vi "Top_Level_Control_v00.vi"() -> ()   [LabVIEW 2010]
uses:
  <vilib>/rvi/interface/nirviCloseFPGA/nirviCloseFPGA.xnode
  <vilib>/rvi/interface/nirviOpenFPGA/nirviOpenFPGA.xnode
  <vilib>/userDefined/High Color/nirio_resource_hc.ctl
  <vilib>/rvi/interface/nirviReadWriteControl/nirviReadWriteControl.xnode
  <vilib>/Utility/error.llb/Error Cluster From Error Code.vi
  <vilib>/rvi/interface/nirviMethod/nirviMethod.xnode
  <vilib>/FPGAPlugInAG/Dynamic/niLvFpga_Close_Dynamic.vi
  NiFpgaLv.dll
  Temporal Clusters Control/FPGA Bitfiles/TemporalClusters_FPGABSlot3_GraphFPGAv07_B46A369A.lvbitx
  Program Files/National Instruments/LabVIEW 2010/Targets/NI/FPGA/StockFPGA_IntfPrivate/ScriptTemplates/StockFPGA_ReadBigControlPlusUnflatten.vi
  Program Files/National Instruments/LabVIEW 2010/Targets/NI/FPGA/StockFPGA_IntfPrivate/ScriptTemplates/StockFPGA_FlattenPlusWriteBigControl.vi
  Program Files/National Instruments/LabVIEW 2010/Targets/NI/FPGA/StockFPGA_IntfPrivate/ScriptTemplates/StockFPGA_InlinedAdjustErrorForReadWrite.vi
  FPGA Bitfiles/PIIphaselocks_FPGATarget_CavitiesPulseFPG_483F4CC6.lvbitx
  <vilib>/FPGAPlugInAG/PXI-7833R/niLvFpga_Open_PXI-7833R.vi
  <vilib>/rvi/ClientSDK/nirviWhatTheDeviceIsDoing.ctl
  <vilib>/rvi/interface/common/dynamic/niFpgaDynamicAddResources.vi
  <vilib>/rvi/errors/niLvFpgaWhatHappensToTopLevelVI.ctl
  <vilib>/rvi/interface/common/niFpgaNodeNameForErrorReporting.ctl
  <vilib>/rvi/errors/niLvFpgaAdjustHostInterfaceError.vi
  Strict Type Defs/Lock or Hold.ctl
  Strict Type Defs/Slider and display.ctl
  Strict Type Defs/I16 white control.ctl
  Strict Type Defs/PII Gains.ctl
  Strict Type Defs/DC polarity.ctl
  Strict Type Defs/Thresh slider.ctl
  Strict Type Defs/I2 gain slider.ctl
  Strict Type Defs/Scan Freq Slider.ctl
  Strict Type Defs/Gains negative vertical.ctl
  Strict Type Defs/Control GUI v01.ctl
  Strict Type Defs/Lock Select.ctl
  Strict Type Defs/Hold All.ctl
  Strict Type Defs/Scope and Safety.ctl
  Strict Type Defs/Pre-Offset.ctl
  Strict Type Defs/Cavity Extras.ctl
  Strict Type Defs/Pulse Control.ctl
  Strict Type Defs/theta.ctl
  Strict Type Defs/Control GUI Graph v00.ctl
  Strict Type Defs/Graph Extras.ctl
  Strict Type Defs/Double Graph control.ctl
  Strict Type Defs/I16 Graph Control.ctl
  Strict Type Defs/GUI HD Graph.ctl
panel:
  out "Any Unlocked?":bool=TRUE
  out "Locked?":T1={"OPO A"=FALSE, "OPO B"=FALSE, "MCC"=FALSE, "Doubler"=TRUE}
  out "Locked?(Graph)":T2={"パラメ A"=TRUE, "パラメ B"=TRUE, "EPR BS"=TRUE, "Graph BS"=TRUE, "HD A"=TRUE, "HD B"=TRUE}
  in  "Measurement OFF":bool
  in  "watertank":bool
  out "Water Tank":dbl(slide)=-0.29411764705882354 scale=-0.3..0.3
  in  "Stop Pulses":bool
  in  "Pulses":bool
  out "Top Loop Count":i32=272090
  out "Measurment Pulse":bool
  out "HD Pulse":bool
  out "Probe OFF Pulse":bool=TRUE
  out "BS Hold Pulse":bool=TRUE
  in  "stop":bool
  in  "Hold All":T3
  in  "Extra Controls":T4(tab)=enum."Other"
  in  "Scope+Safety":T5={"Safety First"={"lim reset"=FALSE, "no limit"=FALSE, "pos slew rate * dt"=12, "neg slew rate * dt"=-12, "Count(Ticks)"=0}, "Scope IPs"={"Trigger Direction"=enum."minus-plus", "Trigger Delay (ms)"=0.0, "Aquisition Rate (kHz)"=4000.0, "Trigger Offset (V)"=0.0, "Scale Offset"={"Scaling"={"Error signal"=1, "Output"=0, "DC Monitor"=1, "Threshold"=1}, "Offset"={"Error Signal"=0, "Output"=0, "DC Monitor"=0, "Threshold"=0}}}}
  in  "Graph Extras":T6={"Error Bit Sh."={"パラメ A"=-2, "パラメ B"=-2, "EPR BS"=0, "Graph BS"=0, "HD A x"=-2, "HD A p"=-2, "HD B x"=-4, "HD B p"=-3}, "I Max value"=2147483647, "I2 Max value"=2147483647, "Scan Offset"={"パラメ A"=0.0, "パラメ B"=0.0, "EPR BS"=0.0, "Graph BS"=0.0, "HD A"=0.0, "HD B"=0.0}, "Scan Ampl."={"パラメ A"=1000.0, "パラメ B"=1000.0, "EPR BS"=1200.0, "Graph BS"=100.0, "HD A"=2000.0, "HD B"=2000.0}, "Scan-PII thresh"={"パラメ A"=100, "パラメ B"=100, "EPR BS"=100, "Graph BS"=100, "Homodyne A"=100, "Homodyne B"=100}, "Re-Scan thresh"={"パラメ A"=1, "パラメ B"=1, "EPR BS"=1, "Graph BS"=1, "Homodyne A"=1, "Homodyne B"=1}, "Post-Offset"={"HD A x"=0.0, "HD A p"=0.0, "HD B x"=0.0, "HD B p"=0.0}}
  in  "Cavity Extras":T9={"Pre-Offset"={"OPO A"=0.0, "OPO B"=0.0, "MCC"=0.0, "Doubler"=0.0}, "Pre-Offset DC"={"OPO A"=0.0, "OPO B"=0.0, "MCC"=0.0, "Doubler"=0.0}, "I Max value"=2147483647, "I2 Max value"=0, "Scan Offset"={"OPO A"=0.0, "OPO B"=0.0, "MCC"=0.0, "Doubler"=0.0}, "Scan Ampl."={"OPO A"=1000.0, "OPO B"=1000.0, "MCC"=1000.0, "Doubler"=1000.0}, "Scan-PII thresh"={"OPO A"=100, "OPO B"=100, "MCC"=100, "Doubler"=100}, "Re-Scan thresh"={"OPO A"=1, "OPO B"=1, "MCC"=4, "Doubler"=0}}
  out "xy HD A":cluster{i16[], i16[]}(graph)
  in  "XY HD ON":bool
  out "xy HD B":cluster{i16[], i16[]}(graph)
  in  "Pulse Control":T11={"BS Hold Invert"=FALSE, "Probe Invert"=FALSE, "HD Invert"=TRUE, "Measurement Invert"=FALSE, "BS Hold Delay"=0, "Probe Delay"=10, "HD Delay"=25, "Measurement delay"=80, "High Pulse"=4000, "Low Pulse"=-3200, "Sample & Hold Period (uSec)"=500, "BS Hold ON until"=325, "Probe OFF until"=315, "HD ON until"=305, "Measurement ON until"=280, "Loop period (us)"=0}
  in  "RMS Thresh":T12={"Pump A"=40, "Pump B"=40, "EPR"=40, "Graph"=40, "HD A"=40, "HD B"=40}
  out "Cavities Pulse Loop count":i32=247262374
  out "Tick Count Cavities (uSec)":u32=4069594290 caption="Cavities Tick Count (uSec)"
  out "Cavities Control Loop count":i32=2147483647
  in  "Safety First Graph":T13={"lim reset"=FALSE, "no limit"=FALSE, "pos slew rate * dt"=40, "neg slew rate * dt"=-40, "Count(Ticks)"=0}
  out "Measurement Tick Count(uSec)":u32=500
  in  "offset time":u32=100
  in  "Measurement OFF (uSec)":u32=1100000
  in  "Inverse (Graph)":bool
  out "PXI Trig 1":bool
  in  "Lock Monitor":T14={"OPO A"=80, "OPO B"=80, "MCC"=80, "Doubler"=0}
  out "PXI Trig 2":bool=TRUE
  out "Cavities error out":errorcluster
  out "Graph error":errorcluster
  in  "Loop Delays (uSec)":u32=5
  in  "Number of Elements":u32=4095
  in  "Cavities_FPGA_v07":T15="RIO0" caption="RIO Device"
  in  "Graph_FPGA_v07":T15="RIO1" caption="RIO Device"
  in  "Scope":T16=TRUE
  out "Scope Graph":cluster{dbl[], dbl[]}[](graph)
  in  "Lock Select":T17
  in  "OPO A":T18={"Offset Error"=-0.004322033898305084, "Gain Error"=1, "Offset DC"=0.18926553672316412, "Gain DC"=1, "P Gain"=12, "P Bit Shift"=-7, "I Bit Shift"=-7, "I2 Bit Shift"=-27, "I Gain"=19, "I2 Gain"=0, "Lock Threshold"=66, "Lock"=FALSE, "Hold"=FALSE, "Scan Frequency"=19, "Scan Bit Shift"=-4, "DC negative"=FALSE, "Gains -ve "=FALSE} {"Scan Frequency" scale=1.0..30.0; "I2 Gain" scale=0.0..10.0; "I Gain" scale=0.0..50.0; "P Gain" scale=0.0..50.0; "Offset DC" scale=-5.0..0.5 scale format="%#_5f"; "Offset Error" scale=-0.01..0.005 scale format="%#_5f"}
  in  "OPO B":T18={"Offset Error"=-0.011977401129943503, "Gain Error"=4, "Offset DC"=1.29177966101695, "Gain DC"=1, "P Gain"=14, "P Bit Shift"=-8, "I Bit Shift"=-8, "I2 Bit Shift"=-27, "I Gain"=13, "I2 Gain"=0, "Lock Threshold"=67, "Lock"=FALSE, "Hold"=FALSE, "Scan Frequency"=10, "Scan Bit Shift"=-5, "DC negative"=TRUE, "Gains -ve "=FALSE} {"Scan Frequency" scale=1.0..30.0; "I2 Gain" scale=0.0..10.0; "I Gain" scale=0.0..50.0; "P Gain" scale=0.0..50.0; "Offset DC" scale=-5.1..3.0 scale format="%#_5f"; "Offset Error" scale format="%#_5f"}
  in  "MCC":T18={"Offset Error"=-0.006610169491525424, "Gain Error"=1, "Offset DC"=0.028813559322033905, "Gain DC"=1, "P Gain"=14, "P Bit Shift"=-8, "I Bit Shift"=-11, "I2 Bit Shift"=-27, "I Gain"=11, "I2 Gain"=0, "Lock Threshold"=20, "Lock"=FALSE, "Hold"=FALSE, "Scan Frequency"=10, "Scan Bit Shift"=-4, "DC negative"=TRUE, "Gains -ve "=TRUE} {"Scan Frequency" scale=1.0..30.0; "I2 Gain" scale=0.0..10.0; "I Gain" scale=0.0..50.0; "P Gain" scale=0.0..50.0; "Offset DC" scale=-0.1..0.2 scale format="%#_5f"; "Offset Error" scale=-0.02..0.01 scale format="%#_5f"}
  in  "Doubler":T18={"Offset Error"=-0.011581920903954804, "Gain Error"=1, "Offset DC"=-0.023163841807909608, "Gain DC"=1, "P Gain"=10, "P Bit Shift"=-7, "I Bit Shift"=-8, "I2 Bit Shift"=-27, "I Gain"=21, "I2 Gain"=0, "Lock Threshold"=12, "Lock"=FALSE, "Hold"=FALSE, "Scan Frequency"=8, "Scan Bit Shift"=-5, "DC negative"=FALSE, "Gains -ve "=FALSE} {"Scan Frequency" scale=1.0..30.0; "I2 Gain" scale=0.0..10.0; "I Gain" scale=0.0..50.0; "P Gain" scale=0.0..50.0; "Offset DC" scale=-0.1..0.1 scale format="%#_5f"; "Offset Error" scale=-0.05..0.05 scale format="%#_5f"}
  in  "パラメ A":T27={"Offset Error"=-0.004689265536723164, "Gain Error"=2, "P Gain"=10, "P Bit Shift"=-7, "I Bit Shift"=-9, "I2 Bit Shift"=-27, "I Gain"=12, "I2 Gain"=0, "Lock Threshold"=13, "Lock"=FALSE, "Hold"=TRUE, "Scan Frequency"=12, "Scan Bit Shift"=-6, "Gains -ve "=FALSE, "Pre- Offset Error"=0.00367231638418079} {"Pre- Offset Error" scale=-0.05..0.05 scale format="%#_5f"; "Scan Frequency" scale=1.0..30.0; "I2 Gain" scale=0.0..10.0; "I Gain" scale=0.0..50.0; "P Gain" scale=0.0..50.0; "Offset Error" scale=-0.01..0.01 scale format="%#_5f"}
  in  "パラメ B":T27={"Offset Error"=0.003389830508474575, "Gain Error"=1, "P Gain"=31, "P Bit Shift"=-8, "I Bit Shift"=-9, "I2 Bit Shift"=-16, "I Gain"=20, "I2 Gain"=3, "Lock Threshold"=13, "Lock"=FALSE, "Hold"=TRUE, "Scan Frequency"=6, "Scan Bit Shift"=-5, "Gains -ve "=FALSE, "Pre- Offset Error"=0.02768361581920904} {"Pre- Offset Error" scale=-0.1..0.1 scale format="%#_5f"; "Scan Frequency" scale=1.0..30.0; "I2 Gain" scale=0.0..10.0; "I Gain" scale=0.0..50.0; "P Gain" scale=0.0..50.0; "Offset Error" scale=-0.04..0.04 scale format="%#_5f"}
  in  "EPR BS":T27={"Offset Error"=-0.0003333333333333334, "Gain Error"=1, "P Gain"=25, "P Bit Shift"=-10, "I Bit Shift"=-10, "I2 Bit Shift"=-17, "I Gain"=22, "I2 Gain"=3, "Lock Threshold"=14, "Lock"=FALSE, "Hold"=TRUE, "Scan Frequency"=9, "Scan Bit Shift"=-6, "Gains -ve "=FALSE, "Pre- Offset Error"=0.011468926553672315} {"Pre- Offset Error" scale=-0.01..0.03 scale format="%#_5f"; "Scan Frequency" scale=1.0..30.0; "I2 Gain" scale=0.0..10.0; "I Gain" scale=0.0..50.0; "P Gain" scale=0.0..50.0; "Offset Error" scale=-0.001..0.001 scale format="%#_5f"}
  in  "Graph BS":T27={"Offset Error"=-0.0011751412429378532, "Gain Error"=1, "P Gain"=12, "P Bit Shift"=-7, "I Bit Shift"=-10, "I2 Bit Shift"=-16, "I Gain"=15, "I2 Gain"=3, "Lock Threshold"=13, "Lock"=FALSE, "Hold"=TRUE, "Scan Frequency"=7, "Scan Bit Shift"=-5, "Gains -ve "=FALSE, "Pre- Offset Error"=0.012796610169491527} {"Pre- Offset Error" scale=-0.005..0.02 scale format="%#_5f"; "Scan Frequency" scale=1.0..30.0; "I2 Gain" scale=0.0..10.0; "I Gain" scale=0.0..50.0; "P Gain" scale=0.0..50.0; "Offset Error" scale format="%#_5f"}
  in  "Homodyne A":T28={"Pre-Offset p Error"=-0.027683615819209043, "Gain Error x"=2, "P Gain"=13, "P Bit Shift"=-10, "I Bit Shift"=-8, "I2 Bit Shift"=-11, "I Gain"=22, "I2 Gain"=2, "Lock Threshold"=28, "Lock"=FALSE, "Hold"=TRUE, "Scan Frequency"=10, "Scan Bit Shift"=-5, "Gains -ve "=FALSE, "Pre- Offset x"=0.02768361581920904, "Lock Angle (θ)"=90.0, "Gain Error p\n\n"=1} {"Lock Angle (θ)" min=-90.0 max=90.0 scale=-90.0..90.0 scale format="%#_2g"; "Pre- Offset x" scale=-0.1..0.1 scale format="%#_5f"; "Scan Frequency" scale=1.0..30.0; "I2 Gain" scale=0.0..10.0; "I Gain" scale=0.0..50.0; "P Gain" scale=0.0..50.0; "Pre-Offset p Error" scale=-0.1..0.1 scale format="%#_5f"}
  in  "Homodyne B":T28={"Pre-Offset p Error"=0.015536723163841807, "Gain Error x"=1, "P Gain"=20, "P Bit Shift"=-6, "I Bit Shift"=-5, "I2 Bit Shift"=-15, "I Gain"=12, "I2 Gain"=3, "Lock Threshold"=15, "Lock"=FALSE, "Hold"=TRUE, "Scan Frequency"=7, "Scan Bit Shift"=-5, "Gains -ve "=TRUE, "Pre- Offset x"=-0.011864406779661014, "Lock Angle (θ)"=90.0, "Gain Error p\n\n"=5} {"Lock Angle (θ)" min=-90.0 max=90.0 scale=-90.0..90.0 scale format="%#_2g"; "Pre- Offset x" scale=-0.1..0.05 scale format="%#_5f"; "Scan Frequency" scale=1.0..30.0; "I2 Gain" scale=0.0..10.0; "I Gain" scale=0.0..50.0; "P Gain" scale=0.0..50.0; "Pre-Offset p Error" scale=-0.05..0.05 scale format="%#_5f"}
  # "All time values are in micro-seconds"
  # "PII Gains"
  # "Lock"
  # "Error Signal"
  # "Monitor"
  # "Scan"
  # "DC positive"
  # "PII Gains"
  # "Lock"
  # "Error Signal"
  # "Monitor"
  # "Scan"
  # "DC positive"
  # "PII Gains"
  # "Lock"
  # "Error Signal"
  # "Monitor"
  # "Scan"
  # "DC positive"
  # "PII Gains"
  # "Lock"
  # "Error Signal"
  # "Monitor"
  # "Scan"
  # "DC positive"
  # "PII Gains"
  # "Lock"
  # "Error Signal"
  # "Scan"
  # "PII Gains"
  # "Lock"
  # "Error Signal"
  # "Scan"
  # "PII Gains"
  # "Lock"
  # "Error Signal"
  # "Scan"
  # "PII Gains"
  # "Lock"
  # "Error Signal"
  # "Scan"
  # "PII Gains"
  # "Lock"
  # "Error Signal"
  # "Scan"
  # "PII Gains"
  # "Lock"
  # "Error Signal"
  # "Scan"
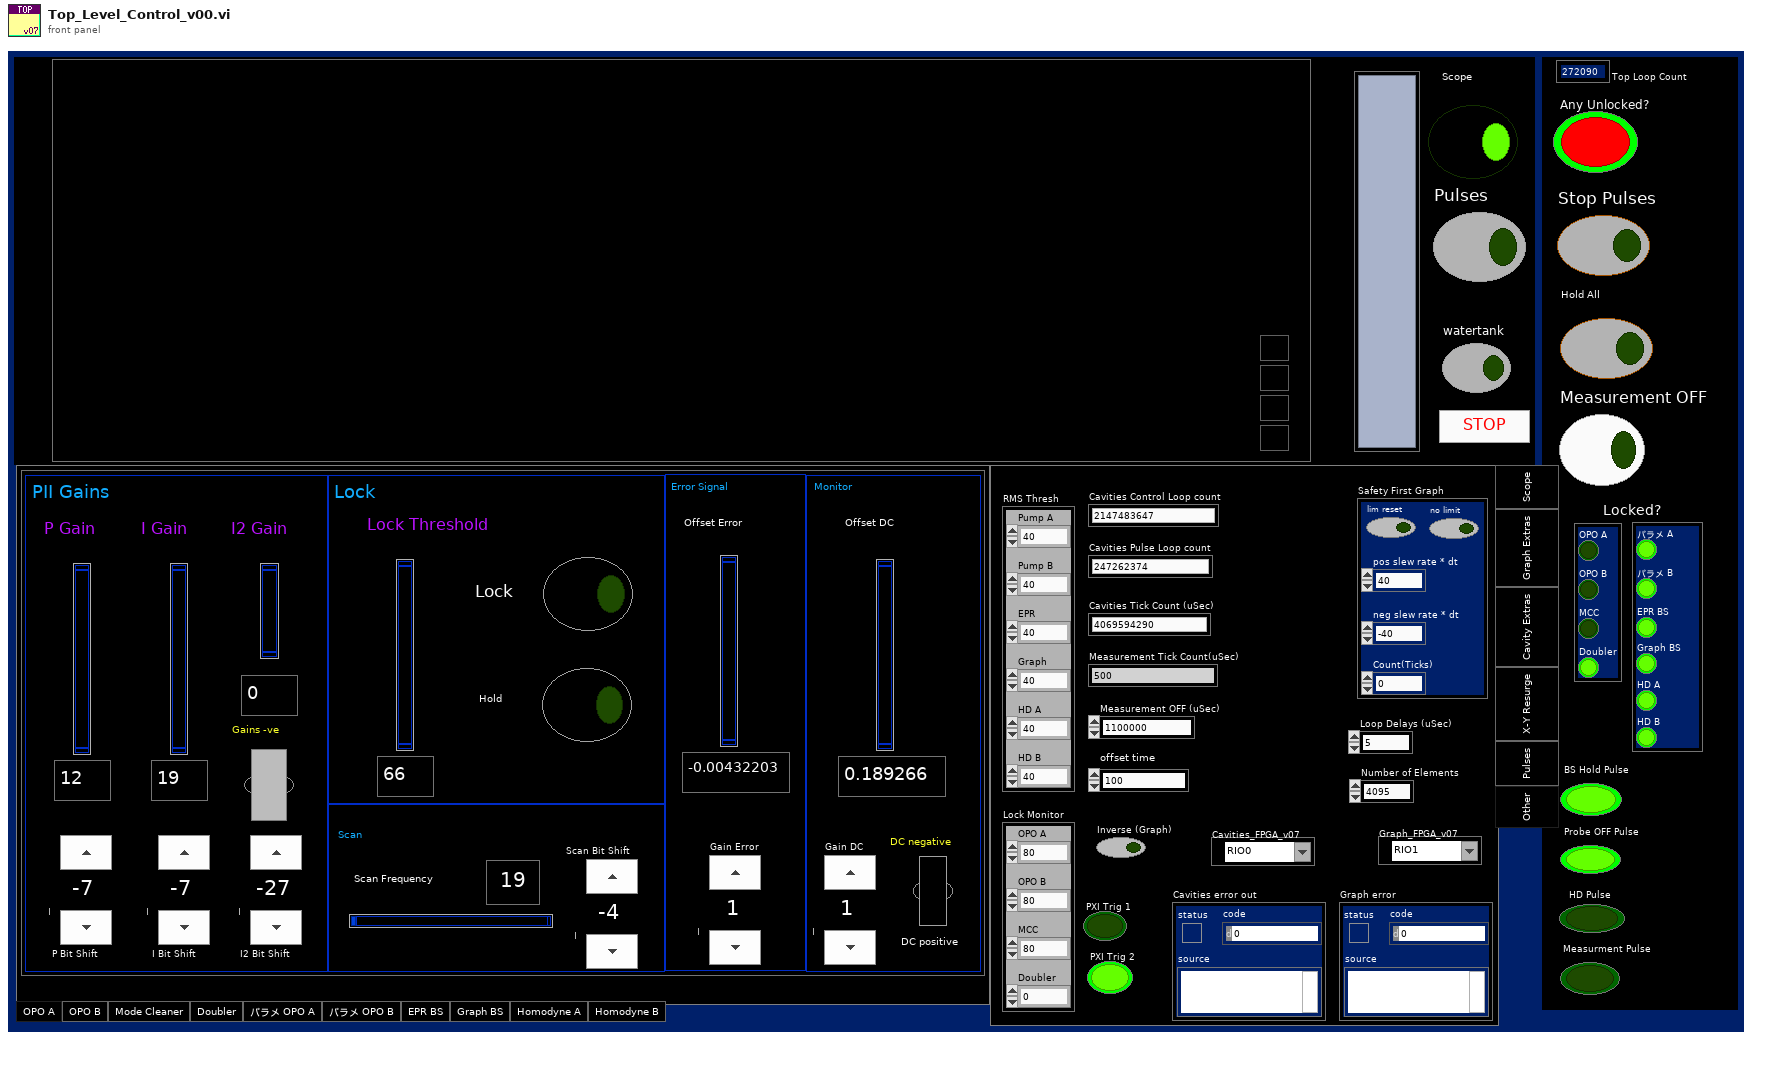
[diagram p1: front panel]
types:
  T1 = cluster{"OPO A":bool, "OPO B":bool, "MCC":bool, "Doubler":bool}
  T2 = cluster{"パラメ A":bool, "パラメ B":bool, "EPR BS":bool, "Graph BS":bool, "HD A":bool, "HD B":bool}
  T3 = typedef "Hold All.ctl" = bool
  T4 = enum32{"Scope", "Graph Extras", "Cavity Extras", "X-Y Resurge", "Pulses", "Other"}
  T5 = typedef "Scope and Safety.ctl" = cluster{"Safety First":cluster{"lim reset":bool, "no limit":bool, "pos slew rate * dt":i16, "neg slew rate * dt":i16, "Count(Ticks)":u32}, "Scope IPs":cluster{"Trigger Direction":enum8{"either", "minus-plus", "plus-minus"}, "Trigger Delay (ms)":dbl, "Aquisition Rate (kHz)":dbl, "Trigger Offset (V)":dbl, "Scale Offset":cluster{"Scaling":cluster{"Error signal":i16, "Output":i16, "DC Monitor":i16, "Threshold":i16}, "Offset":cluster{"Error Signal":i16, "Output":i16, "DC Monitor":i16, "Threshold":i16}}}}
  T6 = typedef "Graph Extras.ctl" = cluster{"Error Bit Sh.":cluster{"パラメ A":i16, "パラメ B":i16, "EPR BS":i16, "Graph BS":i16, "HD A x":i16, "HD A p":i16, "HD B x":i16, "HD B p":i16}, "I Max value":i32, "I2 Max value":i32, "Scan Offset":T7, "Scan Ampl.":T7, "Scan-PII thresh":T8, "Re-Scan thresh":T8, "Post-Offset":cluster{"HD A x":dbl, "HD A p":dbl, "HD B x":dbl, "HD B p":dbl}}
  T7 = typedef "Double Graph control.ctl" = cluster{"パラメ A":dbl, "パラメ B":dbl, "EPR BS":dbl, "Graph BS":dbl, "HD A":dbl, "HD B":dbl}
  T8 = typedef "I16 Graph Control.ctl" = cluster{"パラメ A":i16, "パラメ B":i16, "EPR BS":i16, "Graph BS":i16, "Homodyne A":i16, "Homodyne B":i16}
  T9 = typedef "Cavity Extras.ctl" = cluster{"Pre-Offset":T10, "Pre-Offset DC":T10, "I Max value":i32, "I2 Max value":i32, "Scan Offset":T10, "Scan Ampl.":T10, "Scan-PII thresh":cluster{"OPO A":i16, "OPO B":i16, "MCC":i16, "Doubler":i16}, "Re-Scan thresh":cluster{"OPO A":i16, "OPO B":i16, "MCC":i16, "Doubler":i16}}
  T10 = typedef "Pre-Offset.ctl" = cluster{"OPO A":dbl, "OPO B":dbl, "MCC":dbl, "Doubler":dbl}
  T11 = typedef "Pulse Control.ctl" = cluster{"BS Hold Invert":bool, "Probe Invert":bool, "HD Invert":bool, "Measurement Invert":bool, "BS Hold Delay":u32, "Probe Delay":u32, "HD Delay":u32, "Measurement delay":u32, "High Pulse":i16, "Low Pulse":i16, "Sample & Hold Period (uSec)":u32, "BS Hold ON until":u32, "Probe OFF until":u32, "HD ON until":u32, "Measurement ON until":u32, "Loop period (us)":u16}
  T12 = cluster{"Pump A":i16, "Pump B":i16, "EPR":i16, "Graph":i16, "HD A":i16, "HD B":i16}
  T13 = cluster{"lim reset":bool, "no limit":bool, "pos slew rate * dt":i16, "neg slew rate * dt":i16, "Count(Ticks)":u32}
  T14 = cluster{"OPO A":i16, "OPO B":i16, "MCC":i16, "Doubler":i16}
  T15 = typedef "nirio_resource_hc.ctl" = tag
  T16 = typedef "Lock or Hold.ctl" = bool
  T17 = typedef "Lock Select.ctl" = enum32{"OPO A", "OPO B", "Mode Cleaner", "Doubler", "パラメ OPO A", "パラメ OPO B", "EPR BS", "Graph BS", "Homodyne A", "Homodyne B"}
  T18 = typedef "Control GUI v01.ctl" = cluster{"Offset Error":T19, "Gain Error":T20, "Offset DC":T19, "Gain DC":T20, "P Gain":T21, "P Bit Shift":T20, "I Bit Shift":T20, "I2 Bit Shift":T20, "I Gain":T21, "I2 Gain":T22, "Lock Threshold":T23, "Lock":T16, "Hold":T16, "Scan Frequency":T24, "Scan Bit Shift":T20, "DC negative":T25, "Gains -ve ":T26}
  T19 = typedef "Slider and display.ctl" = dbl
  T20 = typedef "I16 white control.ctl" = i16
  T21 = typedef "PII Gains.ctl" = i32
  T22 = typedef "I2 gain slider.ctl" = i32
  T23 = typedef "Thresh slider.ctl" = i16
  T24 = typedef "Scan Freq Slider.ctl" = u16
  T25 = typedef "DC polarity.ctl" = bool
  T26 = typedef "Gains negative vertical.ctl" = bool
  T27 = typedef "Control GUI Graph v00.ctl" = cluster{"Offset Error":T19, "Gain Error":T20, "P Gain":T21, "P Bit Shift":T20, "I Bit Shift":T20, "I2 Bit Shift":T20, "I Gain":T21, "I2 Gain":T22, "Lock Threshold":T23, "Lock":T16, "Hold":T16, "Scan Frequency":T24, "Scan Bit Shift":T20, "Gains -ve ":T26, "Pre- Offset Error":T19}
  T28 = typedef "GUI HD Graph.ctl" = cluster{"Pre-Offset p Error":T19, "Gain Error x":T20, "P Gain":T21, "P Bit Shift":T20, "I Bit Shift":T20, "I2 Bit Shift":T20, "I Gain":T21, "I2 Gain":T22, "Lock Threshold":T23, "Lock":T16, "Hold":T16, "Scan Frequency":T24, "Scan Bit Shift":T20, "Gains -ve ":T26, "Pre- Offset x":T19, "Lock Angle (θ)":T29, "Gain Error p\n\n":T20}
  T29 = typedef "theta.ctl" = dbl
  T30 = typedef "niFpgaNodeNameForErrorReporting.ctl" = enum16{"Open FPGA VI Reference", "Read/Write Control", "Invoke Method: Abort", "Invoke Method: Acknowledge IRQ", "Invoke Method: Download", "Invoke Method: FIFO.Configure", "Invoke Method: FIFO.Read", "Invoke Method: FIFO.Start", "Invoke Method: FIFO.Stop", "Invoke Method: FIFO.Write", "Invoke Method: Reset", "Invoke Method: Run", "Invoke Method: Wait on IRQ", "Close FPGA VI Reference"}
  T31 = typedef "niLvFpgaWhatHappensToTopLevelVI.ctl" = enum16{"top level VI scripted behind XNode", "top level VI inlined behind XNode"}
  T32 = typedef "Top Level Control.ctl" = cluster{"Safety First":T33, "Error scale":T34, "Lock Select":enum32{"OPO A", "OPO B", "Mode Cleaner", "Doubler", "パラメ OPO A", "パラメ OPO B", "EPR Beamsplitter", "Graph Beamsplitter", "Homodyne A", "Homodyne B"}, "Controls":cluster{"OPO A":T35, "OPO B":T35, "MCC":T35, "Doubler":T35}, "Scope IPs":cluster{"Trigger Direction":enum8{"either", "minus-plus", "plus-minus"}, "Trigger Delay (ms)":dbl, "Aquisition Rate (kHz)":dbl, "Trigger Offset (V)":dbl, "Trigger Channel":i32, "Channel Selector":cluster{"Channel 1":i32, "Channel 2":i32, "Channel 3":i32, "Channel 4":i32}, "Scale Offset":cluster{"Scaling":cluster{"Scan Scale":i16, "Scan Scale 2":i16, "Scan Scale 3":i16, "Scan Scale 4":i16}, "Offset":cluster{"Scan Offset":i16, "Scan Offset 2":i16, "Scan Offset 3":i16, "Scan Offset 4":i16}}}, "PII A":T40, "PII B":T40, "PII MCC":T40, "PII Doubler":T40, "Peak Depth (%)":cluster{"Peak Depth (%) 1":i16, "Peak Depth (%) 2":i16, "Peak Depth (%) 3":i16, "Peak Depth (%) 4":i16}}
  T33 = typedef "Safety First.ctl" = cluster{"lim reset":bool, "no limit":bool, "pos slew rate * dt":i16, "neg slew rate * dt":i16, "Hold All":bool, "Count(Ticks)":u32}
  T34 = typedef "Error_Scale.ctl" = cluster{"Bit Shift":cluster{"Bit Shift 1":i16, "Bit Shift 2":i16, "Bit Shift 3":i16, "Bit Shift 4":i16, "Bit Shift 5":i16, "Bit Shift 6":i16, "Bit Shift 7":i16, "Bit Shift 8":i16}, "Pre-Offset":cluster{"Pre-Offset 1":i16, "Pre-Offset 2":i16, "Pre-Offset 3":i16, "Pre-Offset 4":i16, "Pre-Offset 5":i16, "Pre-Offset 6":i16, "Pre-Offset 7":i16, "Pre-Offset 8":i16}, "Post-Offset ":cluster{"Offset 1":i16, "Offset 2":i16, "Offset 3":i16, "Offset 4":i16, "Offset 5":i16, "Offset 6":i16, "Offset 7":i16, "Offset 8":i16}, "Gains":cluster{"Gain 1":i16, "Gain 2":i16, "Gain 3":i16, "Gain 4":i16, "Gain 5":i16, "Gain 6":i16, "Gain 7":i16, "Gain 8":i16}, "Polarity DC":cluster{"False 1":bool, "False 2":bool, "False 3":bool, "False 4":bool, "DC x -1":bool, "DC x -1 2":bool, "DC x -1 3":bool, "DC x -1 4":bool}}
  T35 = typedef "Control GUI v00.ctl" = cluster{"Pre Offset":T19, "Offset":T19, "Gain":T20, "Bit Shift":T20, "Pre Offset 2":T19, "Offset 2":T19, "Gain 2":T20, "Bit Shift 2":T20, "P Gain":T21, "P Bit Shift":T20, "I Bit Shift":T20, "I2 Bit Shift":T20, "I Gain":T21, "I2 Gain":T21, "Lock Threshold":T23, "Lock":T16, "Hold":T16, "Scan Offset (mV)":T36, "Scan Amplitude (mV)":T36, "Scan Frequency":T37, "Scan Bit Shift":T20, "DC x -1":T25, "Gains x -1":T38, "I Max value":T39, "I2 Max value":T39}
  T36 = typedef "Scan Amp slider.ctl" = dbl
  T37 = typedef "Scan Frequency.ctl" = u16
  T38 = typedef "Gains negative.ctl" = bool
  T39 = typedef "I max value.ctl" = i16
  T40 = typedef "Top Level PII.ctl" = cluster{"Lock":bool, "Hold":bool, "P Gain":i16, "P BS":i16, "I Gain":i16, "I BS":i16, "I2 G":i16, "I2 BS":i16, "Scan Amp":i16, "Scan Off":i16, "Scan FS":u16, "SFS BS":i16, "I Max value":i16, "I2 Max value":i16}
  T41 = cluster{"Trigger Direction":enum8{"either", "minus-plus", "plus-minus"}, "Trigger Delay (ms)":dbl, "Aquisition Rate (kHz)":dbl, "Trigger Offset (V)":dbl, "Scale Offset":cluster{"Scaling":cluster{"Scan Scale":i16, "Scan Scale 2":i16, "Scan Scale 3":i16, "Scan Scale 4":i16}, "Offset":cluster{"Scan Offset":i16, "Scan Offset 2":i16, "Scan Offset 3":i16, "Scan Offset 4":i16}}}
  T42 = cluster{"PII In 1":cluster{"Lock":bool, "Hold":bool, "P Gain":i32, "P BS":i16, "I Gain":i32, "I BS":i16, "I2 G":i32, "I2 BS":i16, "Scan Amp":i16, "Scan Off":i16, "Scan FS":u16, "SFS BS":i16, "I Max value":i32, "I2 Max value":i32, "Scope.Offset":i16, "Trigger Direction":enum8{"either", "minus-plus", "plus-minus"}, "Scan-PII thresh":i16}, "PII In 2":cluster{"Lock":bool, "Hold":bool, "P Gain":i32, "P BS":i16, "I Gain":i32, "I BS":i16, "I2 G":i32, "I2 BS":i16, "Scan Amp":i16, "Scan Off":i16, "Scan FS":u16, "SFS BS":i16, "I Max value":i32, "I2 Max value":i32, "Scope.Offset":i16, "Trigger Direction":enum8{"either", "minus-plus", "plus-minus"}, "Scan-PII thresh":i16}, "PII In 3":cluster{"Lock":bool, "Hold":bool, "P Gain":i32, "P BS":i16, "I Gain":i32, "I BS":i16, "I2 G":i32, "I2 BS":i16, "Scan Amp":i16, "Scan Off":i16, "Scan FS":u16, "SFS BS":i16, "I Max value":i32, "I2 Max value":i32, "Scope.Offset":i16, "Trigger Direction":enum8{"either", "minus-plus", "plus-minus"}, "Scan-PII thresh":i16}, "PII In 4":cluster{"Lock":bool, "Hold":bool, "P Gain":i32, "P BS":i16, "I Gain":i32, "I BS":i16, "I2 G":i32, "I2 BS":i16, "Scan Amp":i16, "Scan Off":i16, "Scan FS":u16, "SFS BS":i16, "I Max value":i32, "I2 Max value":i32, "Scope.Offset":i16, "Trigger Direction":enum8{"either", "minus-plus", "plus-minus"}, "Scan-PII thresh":i16}, "Safety First":cluster{"lim reset":bool, "no limit":bool, "pos slew rate * dt":i16, "neg slew rate * dt":i16, "Hold All":bool, "Count(Ticks)":u32}, "Error scale":cluster{"Pre-Offset":cluster{"Pre-Offset 1":i16, "Pre-Offset 2":i16, "Pre-Offset 3":i16, "Pre-Offset 4":i16, "Pre-Offset 5":i16, "Pre-Offset 6":i16, "Pre-Offset 7":i16, "Pre-Offset 8":i16}, "Post-Offset ":cluster{"Offset 1":i16, "Offset 2":i16, "Offset 3":i16, "Offset 4":i16, "Offset 5":i16, "Offset 6":i16, "Offset 7":i16, "Offset 8":i16}, "Gains":cluster{"Gain 1":i16, "Gain 2":i16, "Gain 3":i16, "Gain 4":i16, "Gain 5":i16, "Gain 6":i16, "Gain 7":i16, "Gain 8":i16}, "Polarity DC":cluster{"False 1":bool, "False 2":bool, "False 3":bool, "False 4":bool, "DC x -1":bool, "DC x -1 2":bool, "DC x -1 3":bool, "DC x -1 4":bool}}, "Lock Thresh":cluster{"OPO A":i16, "OPO B":i16, "MCC":i16, "Doubler":i16}, "Re-Scan Thresh":cluster{"OPO A":i16, "OPO B":i16, "MCC":i16, "Doubler":i16}}
  T43 = typedef "PII individual.ctl" = cluster{"Lock":bool, "Hold":bool, "P Gain":i32, "P BS":i16, "I Gain":i32, "I BS":i16, "I2 G":i32, "I2 BS":i16, "Scan Amp":i16, "Scan Off":i16, "Scan FS":u16, "SFS BS":i16, "I Max value":i32, "I2 Max value":i32, "Scope.Offset":i16, "Trigger Direction":enum8{"either", "minus-plus", "plus-minus"}, "Scan-PII thresh":i16}
  T44 = typedef "Error Scale Graph.ctl" = cluster{"Pre-Offset":cluster{"Pre-Offset 1":i16, "Pre-Offset 2":i16, "Pre-Offset 3":i16, "Pre-Offset 4":i16, "Pre-Offset 5":i16, "Pre-Offset 6":i16, "Pre-Offset 7":i16, "Pre-Offset 8":i16}, "Post-Offset ":cluster{"Offset 1":i16, "Offset 2":i16, "Offset 3":i16, "Offset 4":i16, "Offset 5":i16, "Offset 6":i16, "Offset 7":i16, "Offset 8":i16}, "Gains":cluster{"Gain 1":i16, "Gain 2":i16, "Gain 3":i16, "Gain 4":i16, "Gain 5":i16, "Gain 6":i16, "Gain 7":i16, "Gain 8":i16}, "Bit Shifts":cluster{"Bit Shift 1":i16, "Bit Shift 2":i16, "Bit Shift 3":i16, "Bit Shift 4":i16, "Bit Shift 5":i16, "Bit Shift 6":i16, "Bit Shift 7":i16, "Bit Shift 8":i16}}
  T45 = typedef "Lock Thresh Graph.ctl" = cluster{"Pump A":i16, "Pump B":i16, "EPR":i16, "Graph":i16, "HD A":i16, "HD B":i16}
  T46 = typedef "Theta graph.ctl" = cluster{"HD A Sin Theta":i32, "HD A Cos Theta":i32, "HD B Sin Theta":i32, "HD B Cos Theta":i32}
  T47 = cluster{"PII In 1":T43, "PII In 2":T43, "PII In 3":T43, "PII In 4":T43, "PII In 5":T43, "PII In 6":T43, "Error scale":T44, "Lock Thresh":T45, "Re-Scan Thresh":T45, "Theta":T46, "Safety First":T33}
  T48 = cluster{"Trigger Direction":enum8{"either", "minus-plus", "plus-minus"}, "Delay":u32, "Aquisition Rate (Ticks)":u32, "Offset":i16, "Channel":i32, "Channel Selector":cluster{"Channel 1":i32, "Channel 2":i32, "Channel 3":i32, "Channel 4":i32}}
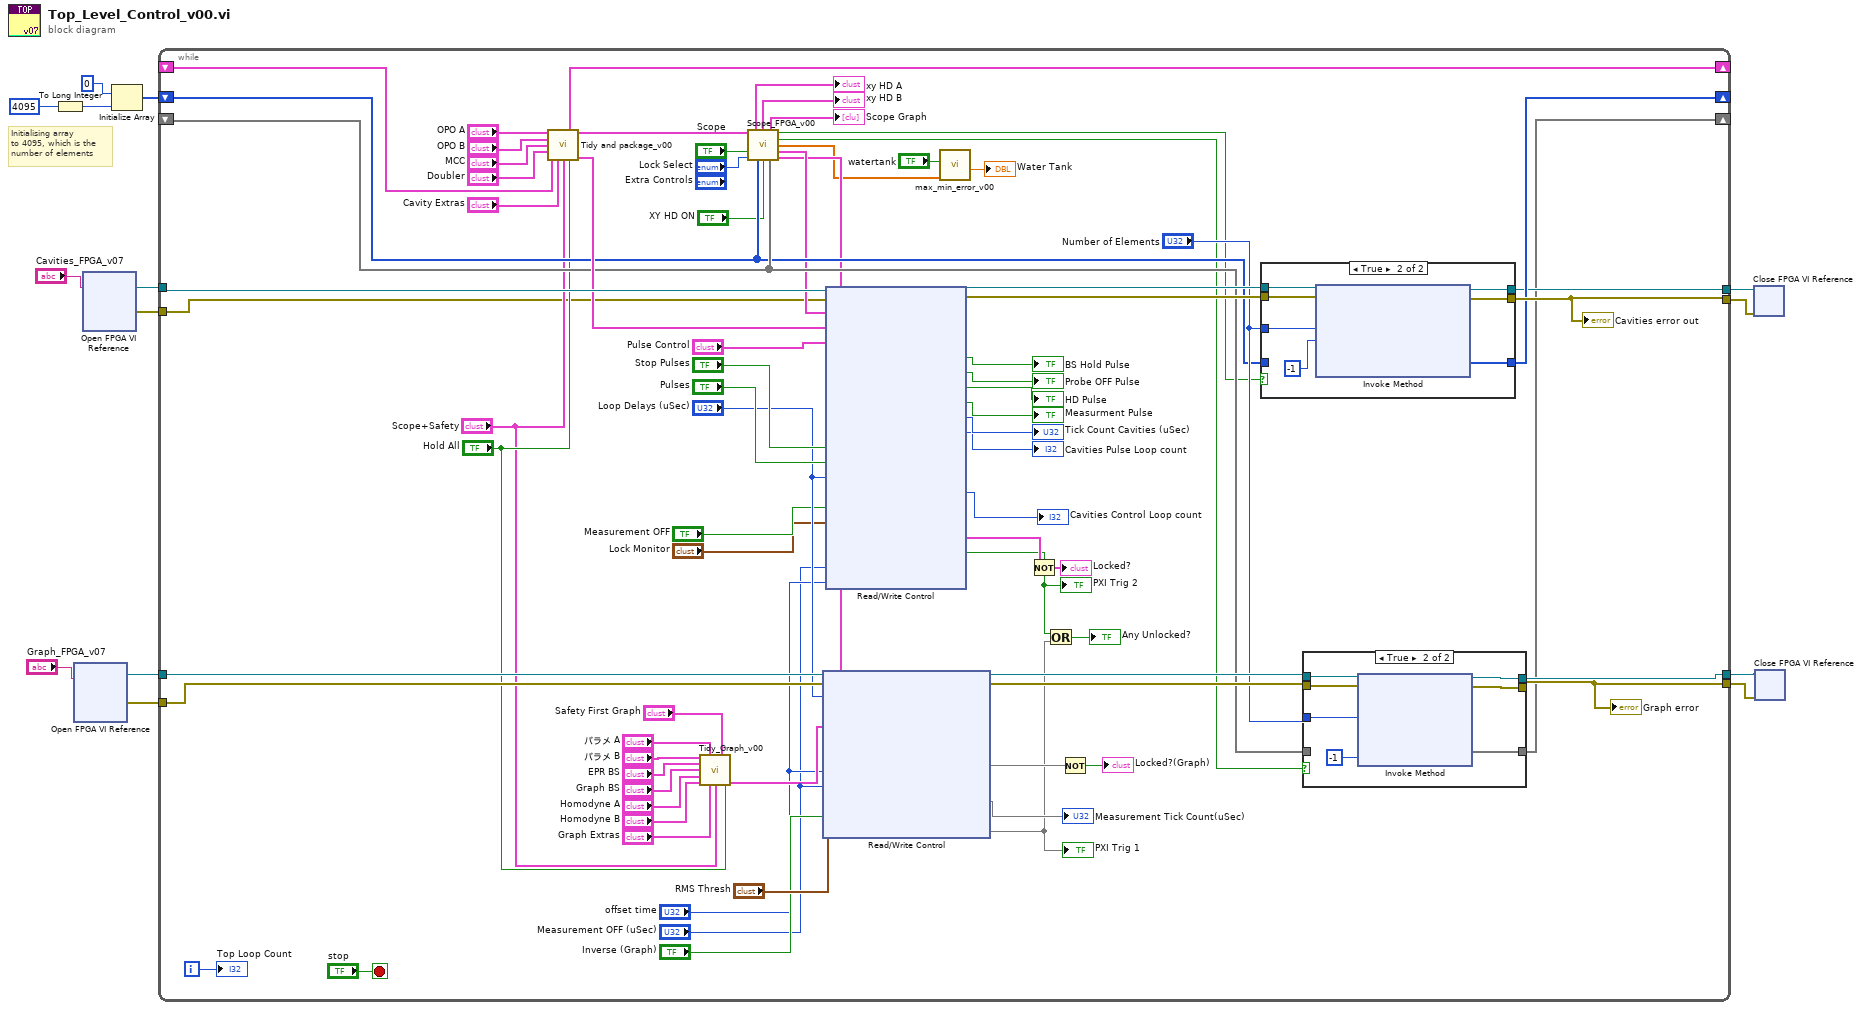
[diagram p0: block diagram]
diagram:
  # "Initialising array\nto 4095, which is the\nnumber of elements"
  n1 = To Long Integer(number=4095) -> (32bit integer=w11:i32)
  n2 = xnode "Open FPGA VI Reference"("resource name"="Graph_FPGA_v07") -> ("FPGA VI Reference Out"=w4:refnum<k20>, "error out"=w3:errorcluster)  [unwired: 1 in]
  n3 = xnode "Open FPGA VI Reference"("resource name"="Cavities_FPGA_v07") -> ("FPGA VI Reference Out"=w13:refnum<k20>, "error out"=w12:errorcluster)  [unwired: 1 in]
  n4 = Initialize Array(u64 0 ("element"), w11) -> (w8:u64[])
  n5 = while {
    tunnel: w13 -> [w91]
    tunnel: w12 -> [w41]
    tunnel: [w87] -> w6
    shift-right: [w85] -> _
    shift-left: w8 -> [w59]
    shift-right: [w81] -> _
    shift-left: _ -> [w78]
    tunnel: [w84] -> w7
    tunnel: w4 -> [w73]
    tunnel: w3 -> [w72]
    tunnel: [w64] -> w2
    tunnel: [w63] -> w1
    shift-right: [w61] -> _
    shift-left: _ -> [w60]
    i -> [w89]
    stop <- "stop" stop-if-true
    n6 = call "Tidy and package_v00.vi"("OPO A"="OPO A", "OPO B"="OPO B", "MCC"="MCC", "Doubler"="Doubler", "PII Controls (-1)"=w78, "Cavity Extras"="Cavity Extras", "Scope+Safety"="Scope+Safety", "Hold All"="Hold All") -> ("PII Controls cluster"=w81:T32, "Scope IPs"=w74:T41, "Control to FPGA"=w77:T42)  [unwired: 5 in]
    n7 = call "Tidy_Graph_v00.vi"("パラメ B"="パラメ B", "パラメ A"="パラメ A", "Safety First Graph"="Safety First Graph", "EPR BS"="EPR BS", "Graph BS"="Graph BS", "Homodyne A"="Homodyne A", "Homodyne B"="Homodyne B", "Graph Extras"="Graph Extras", "Scope+Safety"="Scope+Safety", "Hold All"="Hold All") -> ("Control Graph to FPGA"=w46:T47)  [unwired: 5 in]
    n8 = call "Scope_FPGA_v00.vi"("Scope IPs"=w74, "Scope"="Scope", "Lock Select"="Lock Select", "Cavities Data"=w59, "XY HD ON"="XY HD ON", "Graph Data"=w60) -> ("xy HD A"=→"xy HD A":cluster{i16[], i16[]}, "xy HD B"=→"xy HD B":cluster{i16[], i16[]}, "Scope OP Graph"=→"Scope Graph":cluster{dbl[], dbl[]}[], "Scope Cavities ON"=w43:bool, "Scope Graph ON"=w42:bool, "error"=w32:dbl[], "Scope Cavities"=w47:T48, "Scope Graph"=w35:T48)  [unwired: 2 in]
    n9 = xnode "Read/Write Control"("FPGA VI Reference In"=w73, "error in"=w72, "Graph Delay(uSec)"="Loop Delays (uSec)", "Scope"=w35, "Control"=w46, "RMS Thresh"="RMS Thresh", "offset time"="offset time", "Measurement OFF (uSec)"="Measurement OFF (uSec)", "Inverse"="Inverse (Graph)") -> ("FPGA VI Reference Out"=w65:refnum<k20>, "error out"=w66:errorcluster, "Unlocked?(T=yes)"=w26, "Measurement Tick Count(uSec)"=→"Measurement Tick Count(uSec)", "PXI Trig 1"=w16)
    "PXI Trig 1" <- w16
    n10 = xnode "Read/Write Control"("FPGA VI Reference In"=w91, "error in"=w41, "Scope"=w47, "Control"=w77, "Pulse Control"="Pulse Control", "stop pulse loop"="Stop Pulses", "Pulse Loop On"="Pulses", "Cavities Delay(uSec)"="Loop Delays (uSec)", "Measurement OFF"="Measurement OFF", "Lock Monitor"="Lock Monitor", "Measurement OFF (uSec)"="Measurement OFF (uSec)", "offset time"="offset time") -> ("FPGA VI Reference Out"=w86:refnum<k20>, "error out"=w88:errorcluster, "BS Hold Pulse"=→"BS Hold Pulse":bool, "Probe OFF Pulse"=→"Probe OFF Pulse":bool, "HD Pulse"=→"HD Pulse":bool, "Measurment Pulse"=→"Measurment Pulse":bool, "Tick Count(uSec)"=→"Tick Count Cavities (uSec)":u32, "Pulse Loop count"=→"Cavities Pulse Loop count":i32, "Control Loop count"=→"Cavities Control Loop count":i32, "Unlocked?(T=yes)"=w21:T1, "PXI Trig 2"=w17:bool)
    "PXI Trig 2" <- w17
    n11 = call "max_min_error_v00.vi"("Array"=w32, "maxmin"="watertank") -> ("x+y"=→"Water Tank":dbl)  [unwired: 7 in, 2 out]
    n12 = Not(x=w21) -> (.not. x?=→"Locked?":T1)
    n13 = Or(x=w17, y=w16) -> (x .or. y?=→"Any Unlocked?":bool)
    n14 = Not(x=w26) -> (.not. x?=→"Locked?(Graph)":bool)
    n15 = case shown="True" w43 {
      tunnel: w88 -> [w243 w250]
      tunnel: [w243 w249] -> w87
      tunnel: w86 -> [w242 w248]
      tunnel: [w242 w247] -> w84
      tunnel: [w241 w246] -> w85
      tunnel: w59 -> [w241 _]
      tunnel: "Number of Elements" -> [_ w244]
      frame False {
      }
      frame True {
        n16 = xnode "Invoke Method"("FPGA VI Reference In"=w248, "error in"=w250, "Number of Elements"=w244, "Timeout (ms)"=-1) -> ("FPGA VI Reference Out"=w247:refnum<k20>, "error out"=w249:errorcluster, "Data"=w246:u64[])  [unwired: 1 out]
      }
    }
    "Cavities error out" <- w87
    n17 = case shown="True" w42 {
      tunnel: w66 -> [w94 w101]
      tunnel: [w94 w100] -> w63
      tunnel: w65 -> [w93 w99]
      tunnel: [w93 w98] -> w64
      tunnel: [w92 w97] -> w61
      tunnel: w60 -> [w92 _]
      tunnel: "Number of Elements" -> [_ w95]
      frame False {
      }
      frame True {
        n18 = xnode "Invoke Method"("FPGA VI Reference In"=w99, "error in"=w101, "Number of Elements"=w95, "Timeout (ms)"=-1) -> ("FPGA VI Reference Out"=w98:refnum<k20>, "error out"=w100:errorcluster, "Data"=w97:void[])  [unwired: 1 out]
      }
    }
    "Graph error" <- w63
    "Top Loop Count" <- w89
  }
  n19 = xnode "Close FPGA VI Reference"("FPGA VI Reference In"=w7, "error in"=w6) -> ()  [unwired: 1 out]
  n20 = xnode "Close FPGA VI Reference"("FPGA VI Reference In"=w2, "error in"=w1) -> ()  [unwired: 1 out]
